vi "Mouse Loop.vi"(0 "Mouse Sensor In":T1) -> (3 "x displacement":i8, 4 "y displacement":i8, 5 "Timed out?":bool)   [LabVIEW 2012, in "Mouse IO.lvlib"]
uses:
  Mouse IO.lvlib
panel:
  out "Mouse Sensor Out":T1
  # "Mouse Interface\n===\nMain data acuisition loop for mouse sensor.\nLoop @ 50Hz and read X & Y displacement.\nSensor will lock and wait for up to 18ms."
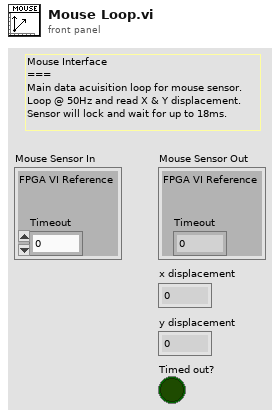
[diagram p1: front panel]
types:
  T1 = cluster{"FPGA VI Reference":refnum<k20>, "Timeout":i32}
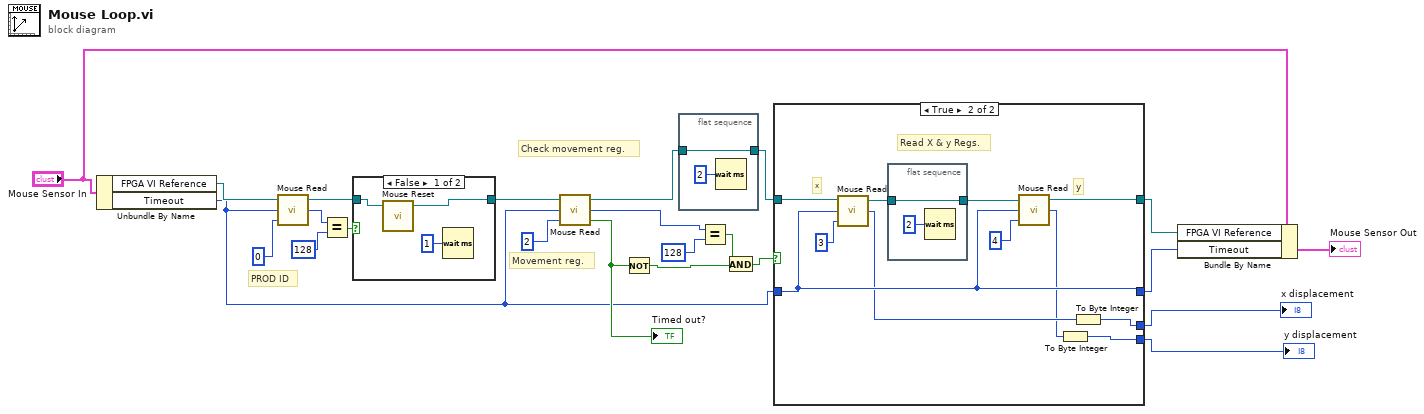
[diagram p0: block diagram]
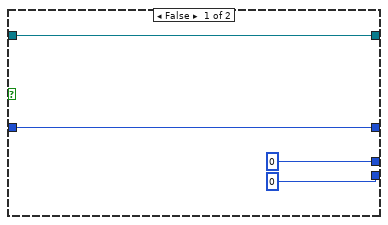
[diagram p3: hidden frame]
diagram:
  # "Check movement reg."
  # "Movement reg."
  # "PROD ID"
  n1 = Unbundle By Name("Mouse Sensor In") -> ("FPGA VI Reference"=w6:refnum<k20>, "Timeout"=w5:i32)
  n2 = call "Mouse Read.vi"("Read Address"=u8 0, "Timeout (ms)"=w5, "FPGA VI Reference In"=w6) -> ("Read Data out"=w11:u8, "FPGA VI Reference Out"=w8:refnum<k20>)  [unwired: 1 out]
  n3 = Equal?(x=w11, y=u8 128) -> (x = y?=w9:bool)
  n4 = case shown="False" w9 {
    tunnel: w8 -> [w26 w27]
    tunnel: [w25 w27] -> w7
    frame False {
      n5 = call "Mouse Reset.vi"("FPGA VI Reference In"=w26) -> ("FPGA VI Reference Out"=w25:refnum<k20>)  [unwired: 3 in, 1 out]
      n6 = Wait (ms)(milliseconds to wait=u32 1) -> ()  [unwired: 1 out]
    }
    frame True {
    }
  }
  n7 = call "Mouse Read.vi"("Read Address"=u8 2, "Timeout (ms)"=w5, "FPGA VI Reference In"=w7) -> ("Timed out?"=w17:bool, "Read Data out"=w15:u8, "FPGA VI Reference Out"=w14:refnum<k20>)
  "Timed out?" <- w17
  n8 = Not(x=w17) -> (.not. x?=w16:bool)
  n9 = flat-sequence {
    tunnel: w14 -> [w29]
    tunnel: [w29] -> w13
    frame #0 {
      n10 = Wait (ms)(milliseconds to wait=u32 2) -> ()  [unwired: 1 out]
    }
  }
  n11 = Equal?(x=w15, y=u8 128) -> (x = y?=w18:bool)
  n12 = And(x=w18, y=w16) -> (x .and. y?=w12:bool)
  n13 = case shown="True" w12 {
    tunnel: w13 -> [w33 w44]
    tunnel: [w33 w43] -> w4
    tunnel: w5 -> [w32 w42]
    tunnel: [w32 w42] -> w3
    tunnel: [i8 0 ("Read Data out") w37] -> w22
    tunnel: [i8 0 ("Read Data out") w36] -> w23
    frame False {
    }
    frame True {
      # "y"
      # "x"
      # "Read X & y Regs."
      n14 = call "Mouse Read.vi"("Read Address"=u8 3, "Timeout (ms)"=w42, "FPGA VI Reference In"=w44) -> ("Read Data out"=w39:u8, "FPGA VI Reference Out"=w35:refnum<k20>)  [unwired: 1 out]
      n15 = flat-sequence {
        tunnel: w35 -> [w46]
        tunnel: [w46] -> w34
        frame #0 {
          n16 = Wait (ms)(milliseconds to wait=u32 2) -> ()  [unwired: 1 out]
        }
      }
      n17 = call "Mouse Read.vi"("Read Address"=u8 4, "Timeout (ms)"=w42, "FPGA VI Reference In"=w34) -> ("Read Data out"=w38:u8, "FPGA VI Reference Out"=w43:refnum<k20>)  [unwired: 1 out]
      n18 = To Byte Integer(number=w38) -> (8bit integer=w36:i8)
      n19 = To Byte Integer(number=w39) -> (8bit integer=w37:i8)
    }
  }
  "x displacement" <- w22
  "y displacement" <- w23
  n20 = Bundle By Name(cluster="Mouse Sensor In", "FPGA VI Reference"=w4, "Timeout"=w3) -> (→"Mouse Sensor Out":T1)
